vi "Test_dynamic-range-adjust.vi"() -> ()   [LabVIEW 2018]
uses:
  <vilib>/vision/NI_Vision_Development_Module.lvlib
panel:
  out "Histogram Graph":T1(graph)
  in  "Slide":cluster{i32, i32}(slide)={0, 4} scale=0.0..65535.0
  in  "Stop":bool
  out "Image":T2(plugin-control)
  in  "File Path":path
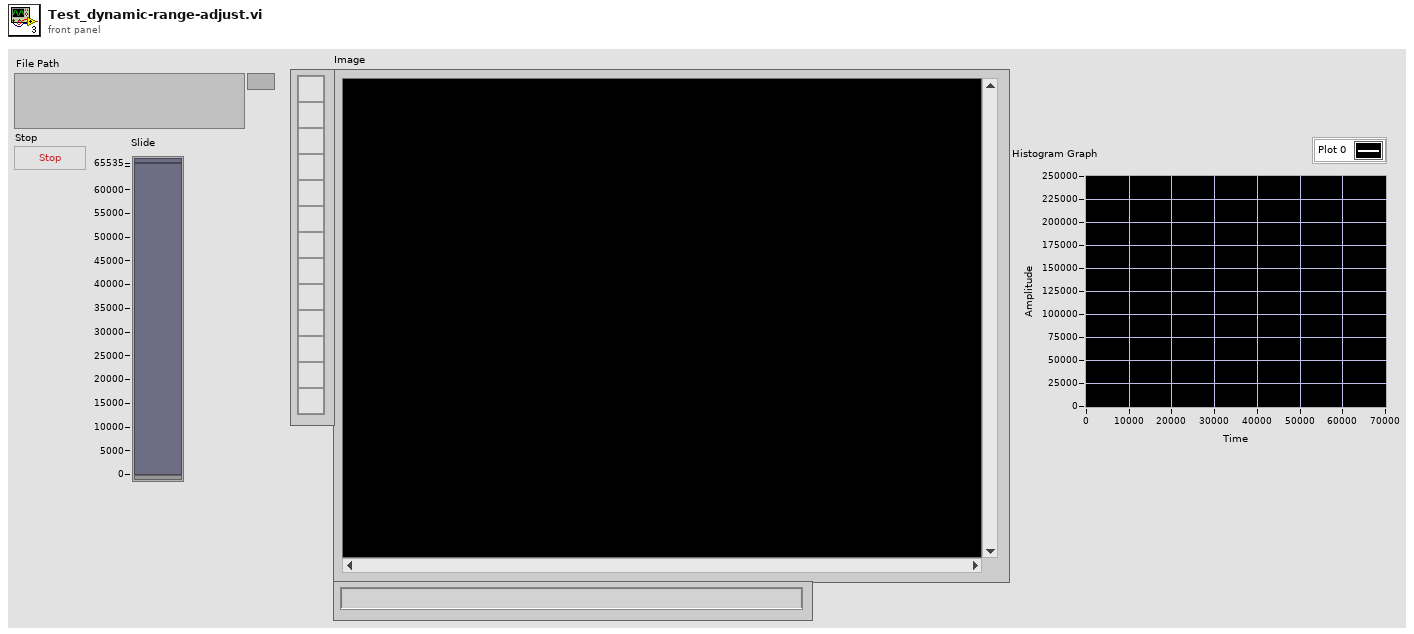
[diagram p1: front panel]
types:
  T1 = cluster{"Starting Value":sgl, "Incremental Value":sgl, "Histogram":u32[]}
  T2 = typedef "IMAQ Image.ctl" = refnum<image>
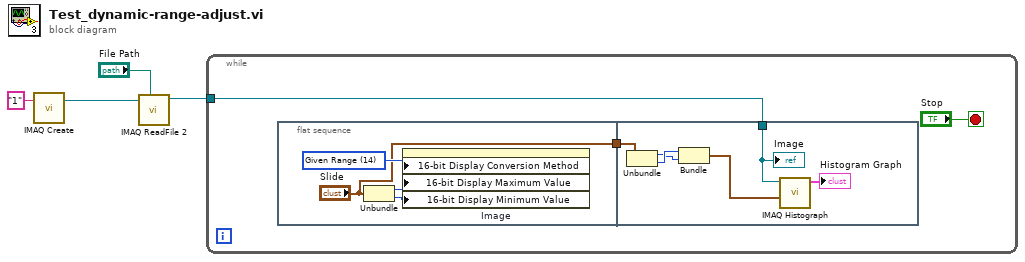
[diagram p0: block diagram]
diagram:
  n1 = call "IMAQ Create"("Image Name"="1") -> ("New Image"=w4:T2)  [unwired: 4 in, 1 out]
  n2 = call "IMAQ ReadFile 2"("File Path"="File Path", "Image"=w4) -> ("Image Out"=w1:T2)  [unwired: 5 in, 4 out]
  n3 = while {
    tunnel: w1 -> [w6]
    stop <- "Stop" stop-if-true
    n4 = flat-sequence {
      tunnel: ["Slide"] -> w5
      tunnel: w6 -> [w17]
      tunnel: w5 -> [w15]
      frame #0 {
        w11 = u32 14 items=["Default"=10, "Most Significant Bits"=11, "Full Dynamic"=12, "Downshift"=13, "Given Range"=14, "90% Dynamic"=15, "Given Percent Range"=16] ("16-bit Display Mapping:Conversion Method")
        n5 = Unbundle("Slide") -> (w10:i32, w9:i32)
        n6 = property on="Image" class="ImageControl"("16-bit Display Conversion Method"=w11, "16-bit Display Maximum Value"=w10, "16-bit Display Minimum Value"=w9) -> ()  [unwired: 2 in, 2 out]
      }
      frame #1 {
        n7 = Unbundle(w15) -> (w13:i32, w14:i32)
        n8 = Bundle(w14, w13) -> (w12:cluster{i32, i32})  [unwired: 1 in]
        n9 = call "IMAQ Histograph"("Interval Range"=w12, "Image"=w17) -> ("Histogram Graph"=→"Histogram Graph":T1)  [unwired: 6 in, 3 out]
        "Image" <- w17
      }
    }
  }
